vi "Initialize Modbus Client Serial.vi"(0 "MODBUS in":refnum<class "Modbus.lvclass">, 1 "protocol (RTU)":enum16{"RTU", "ASCII", "TCP"}(ring), 2 "station address (1)":u8=1, 3 "timeout, ms (300)":u32=300, 5 "port":refnum<visa-resource-name>, 7 "baud rate (9600)":u32=9600, 9 "data bits (8)":u16=8, 11 "error in (no error)":errorcluster, 12 "parity (even)":enum16{"None", "Odd", "Even", "Mark", "Space"}(ring)=enum."Even", 13 "stop bits (1.0)":u16(ring)=10 items=["1.0"=10, "1.5"=15, "2.0"=20], 14 "flow control (none)":u16(ring) items=["None", "XON/XOFF", "RTS/CTS", "XON/XOFF & RTS/CTS", "DTR/DSR", "XON/XOFF & DTR/DSR"]) -> (4 "MODBUS Out":refnum<class "Modbus.lvclass">, 15 "error out":errorcluster)   [LabVIEW 2020, in "Library Instrument & Equipement.lvlib" / "Library Relay_Board.lvlib" / "Modbus.lvclass"]
doc: "Initializes serial connection to Modbus server using specified settings."
uses:
  Modbus.lvclass
  Modbus.lvclass/Modbus.ctl
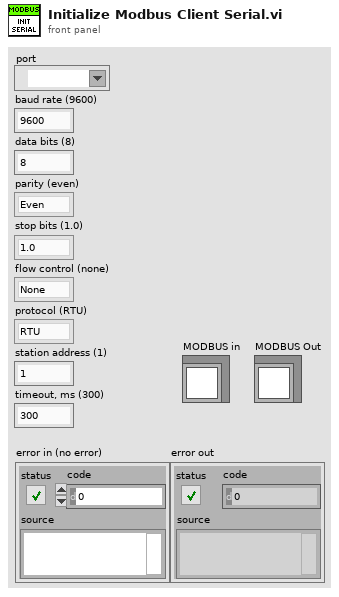
[diagram p1: front panel]
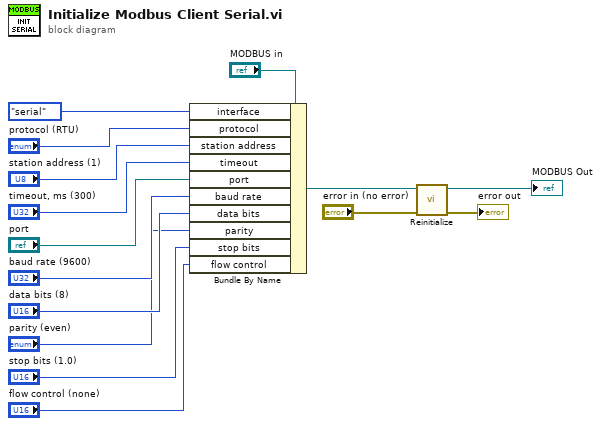
[diagram p0: block diagram]
diagram:
  n1 = Bundle By Name(cluster="MODBUS in", "interface"=enum16{"serial", "network"}."serial" ("mode"), "protocol"="protocol (RTU)", "station address"="station address (1)", "timeout"="timeout, ms (300)", "port"="port", "baud rate"="baud rate (9600)", "data bits"="data bits (8)", "parity"="parity (even)", "stop bits"="stop bits (1.0)", "flow control"="flow control (none)") -> (w14:refnum<class "Modbus.lvclass">)
  n2 = call "Reinitialize.vi"("error in (no error)"="error in (no error)", "MODBUS in"=w14) -> ("error out"=→"error out":errorcluster, "MODBUS Out"=→"MODBUS Out":refnum<class "Modbus.lvclass">)  [unwired: 8 in]
